vi "Init (Instance).vi"(8 "error in (no error)":errorcluster, 10 "Close previous? [T]":bool=TRUE, 11 "Carya Config (By Reference).lvclass":refnum<class "Carya Config (By Reference).lvclass">) -> (0 "error out":errorcluster, 1 "Name":string, 2 "New":bool=TRUE, 3 "Carya Config (Buffer) out":refnum<class "CConfig By Ref Buffer.lvclass">)   [LabVIEW 2013, in "CConfig By Ref Buffer.lvclass"]
doc: "Copyright 2018, Carya Automatisering, Wiebe Walstra."
uses:
  CConfig By Ref Buffer.lvclass
  Carya Config (By Reference).lvclass
  Buffer Functions.ctl
  CConfig By Ref Buffer.lvclass/CConfig By Ref Buffer.ctl
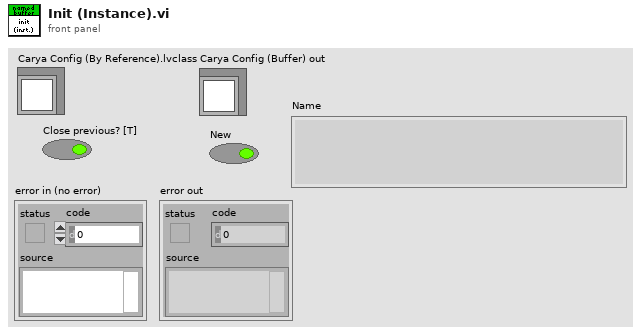
[diagram p1: front panel]
types:
  T1 = typedef "CConfig By Ref Buffer.lvclass/Buffer Functions.ctl" = enum16{"register", "get and lock", "set and unlock", "unlock", "unregister", "check"}
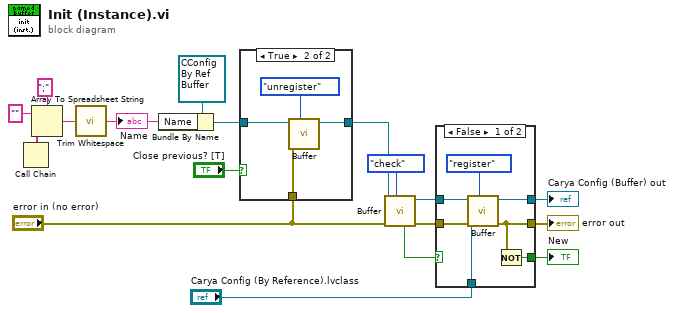
[diagram p0: block diagram]
diagram:
  n1 = Call Chain() -> (call chain=w10:string[])
  n2 = Array To Spreadsheet String(delimiter (Tab)=";" ("spreadsheet string"), array=w10, 3:"" ("format string")) -> (spreadsheet string=w7:string)
  n3 = call <vilib>:"Trim Whitespace.vi"("string"=w7) -> ("trimmed string"=w6:string)  [unwired: 1 in]
  "Name" <- w6
  n4 = Bundle By Name(cluster=refnum<class "CConfig By Ref Buffer.lvclass"> refnum ("Carya Config (Buffer) in"), "Name"=w6) -> (w5:refnum<class "CConfig By Ref Buffer.lvclass">)
  n5 = case shown="True" "Close previous? [T]" {
    tunnel: w5 -> [w19 w22]
    tunnel: [w19 w21] -> w4
    tunnel: "error in (no error)" -> [_ w20]
    frame False {
    }
    frame True {
      n6 = call "Buffer.vi"("Functions"=Buffer_Functions."unregister", "error in (no error)"=w20, "Carya Config (Buffer) in"=w22) -> ("Carya Config (Buffer) out"=w21:refnum<class "CConfig By Ref Buffer.lvclass">)  [unwired: 4 in, 4 out]
    }
  }
  n7 = call "Buffer.vi"("Functions"=Buffer_Functions."check", "error in (no error)"="error in (no error)", "Carya Config (Buffer) in"=w4) -> ("error out"=w14:errorcluster, "Carya Config (Buffer) out"=w15:refnum<class "CConfig By Ref Buffer.lvclass">, "Wait\\Check"=w13:bool)  [unwired: 4 in, 2 out]
  n8 = case shown="False" w13 {
    tunnel: [w30 w32] -> w18
    tunnel: w15 -> [w28 w32]
    tunnel: w14 -> [w27 w31]
    tunnel: [w26 w31] -> w12
    tunnel: [w25 _] -> w11
    tunnel: "Carya Config (By Reference).lvclass" -> [w24 _]
    frame False {
      n9 = call "Buffer.vi"("Functions"=Buffer_Functions."register", "error in (no error)"=w27, "Config in"=w24, "Carya Config (Buffer) in"=w28) -> ("error out"=w26:errorcluster, "Carya Config (Buffer) out"=w30:refnum<class "CConfig By Ref Buffer.lvclass">)  [unwired: 3 in, 3 out]
      n10 = Not(x=w26) -> (.not. x?=w25:bool)
    }
    frame True {
    }
  }
  "error out" <- w12
  "Carya Config (Buffer) out" <- w18
  "New" <- w11
